vi "Read Button.vi"(8 "error in (no error)":errorcluster, 11 "ControlMouseUpMsg in":refnum<class "ControlMouseUpMsg.lvclass">) -> (0 "error out":errorcluster, 2 "Button":u16, 3 "ControlMouseUpMsg out":refnum<class "ControlMouseUpMsg.lvclass">)   [LabVIEW 2015, in "ActorEvents.lvlib" / "ControlMouseUpMsg.lvclass"]
uses:
  ControlMouseUpMsg.lvclass
  ControlMouseUpMsg.lvclass/ControlMouseUpMsg.ctl
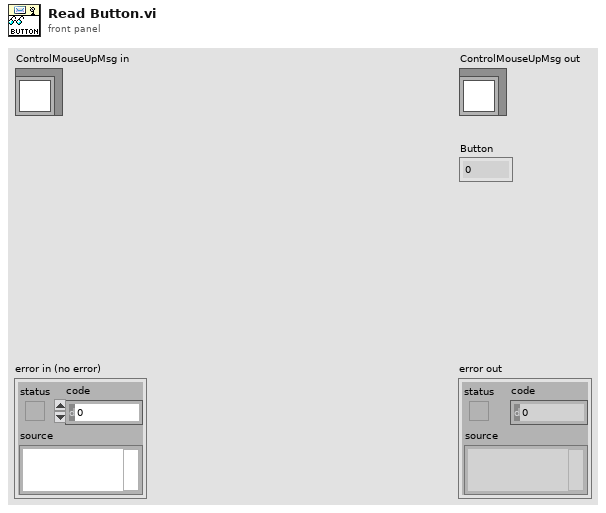
[diagram p1: front panel]
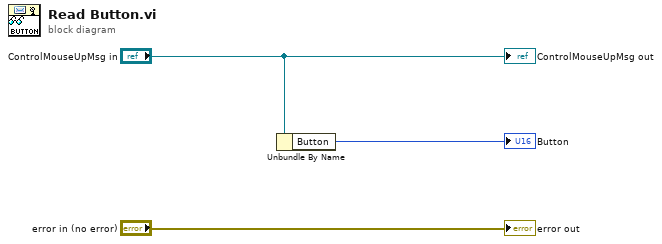
[diagram p0: block diagram]
diagram:
  n1 = Unbundle By Name("ControlMouseUpMsg in") -> ("Button"=→"Button":u16)
  "error out" <- "error in (no error)"
  "ControlMouseUpMsg out" <- "ControlMouseUpMsg in"
